vi "SLM.vi"() -> ()   [LabVIEW 2019]
uses:
  PCIe16LabVIEWSDK/Interface.dll
panel:
  out "Phase Image":u16[][](array[numeric])
  out "SLM":bool
  in  "Start SLM":bool
  out "Update SLM":bool
  out "PCIe16SDK Path":string
  out "Board ID":i32
  out "# of Boards":i32
  in  "SLM Image Path":path
  out "SLM Image":T1(plugin-control)
  out "Init.":bool
  in  "Stop":bool
types:
  T1 = typedef "IMAQ Image.ctl" = refnum<image>
  T2 = typedef "Image Type" = u32
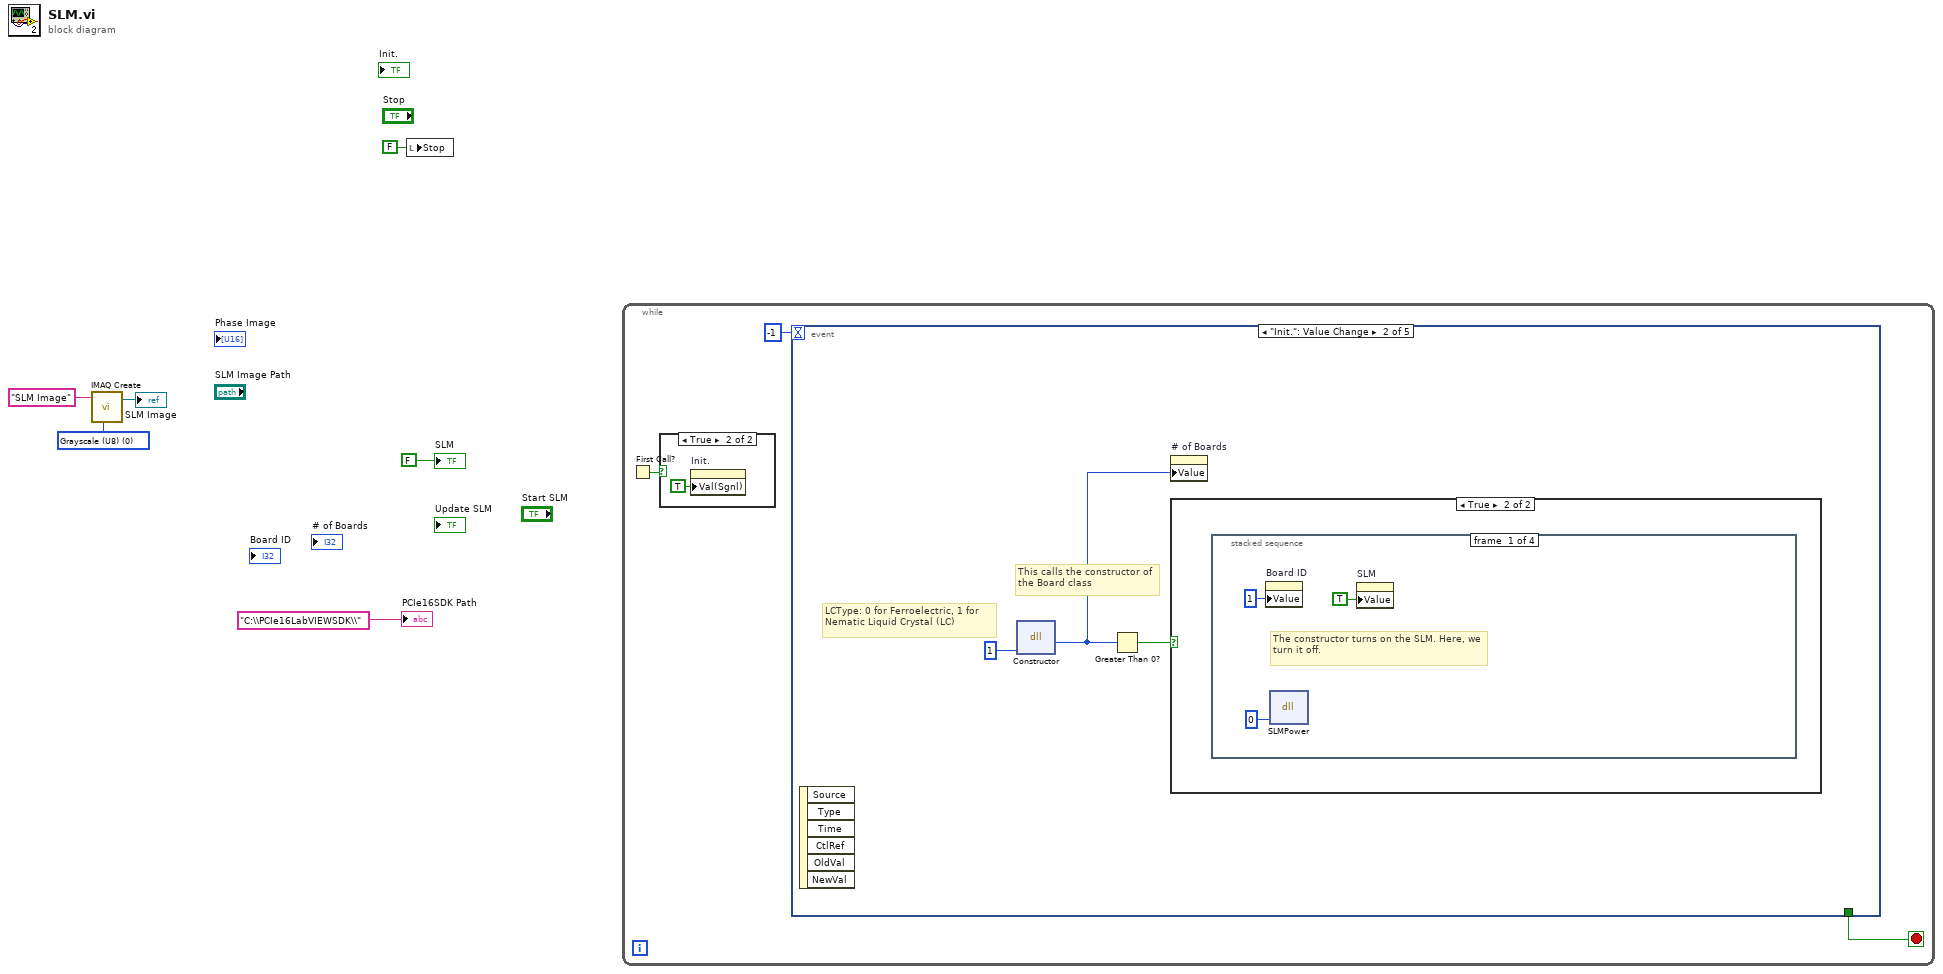
[diagram p0: block diagram]
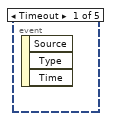
[diagram p3: hidden frame]
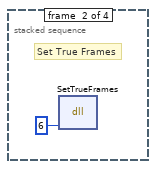
[diagram p5: hidden frame]
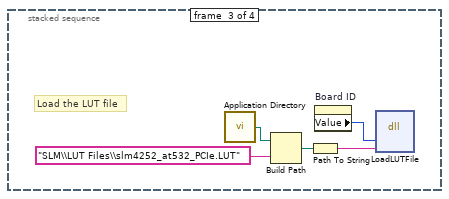
[diagram p6: hidden frame]
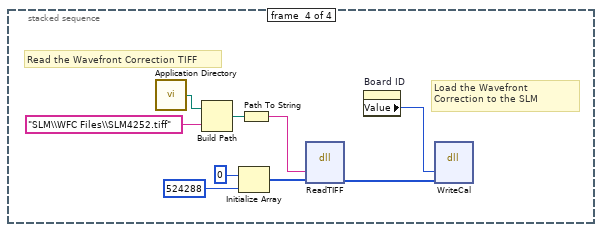
[diagram p7: hidden frame]
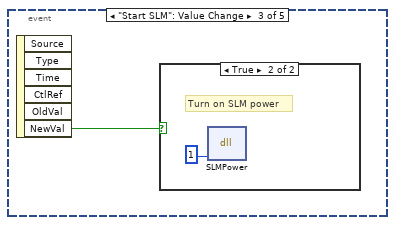
[diagram p8: hidden frame]
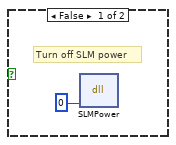
[diagram p9: hidden frame]
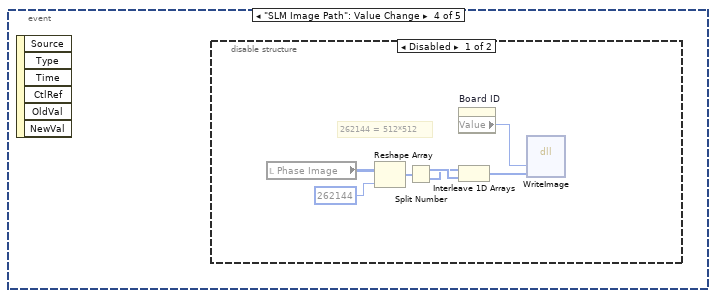
[diagram p10: hidden frame]
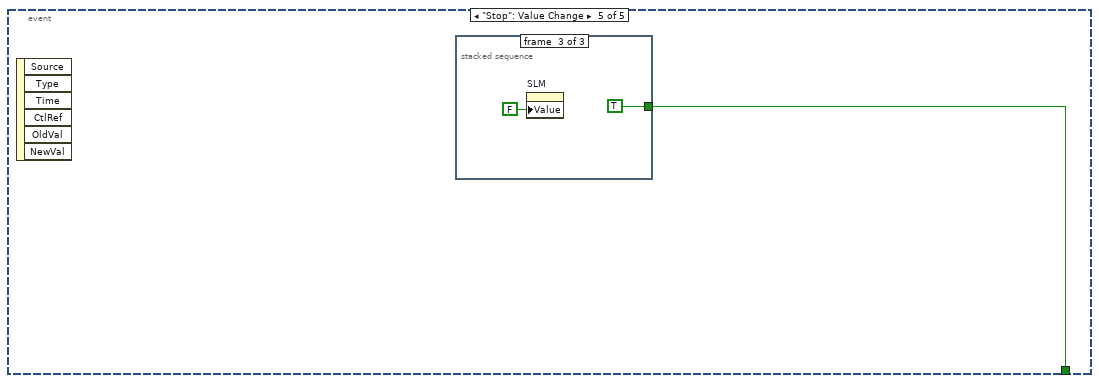
[diagram p12: hidden frame]
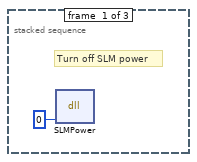
[diagram p13: hidden frame]
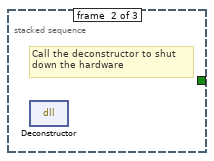
[diagram p14: hidden frame]
diagram:
  w3 = T2 0 items=["Grayscale (U8)", "Grayscale (I16)", "Grayscale (SGL)", "Complex (CSG)", "RGB (U32)", "HSL (U32)", "RGB (U64)", "Grayscale (U16)"] ("Image Type")
  n1 = call "IMAQ Create"("Image Name"="SLM Image", "Image Type"=w3) -> ("New Image"=→"SLM Image":T1)  [unwired: 3 in, 1 out]
  n2 = local write "Stop"(FALSE ("Stop")) -> ()
  n3 = while {
    stop <- w8 stop-if-true
    n4 = First Call?() -> (First Call?: T/F=w7:bool)
    n5 = case shown="True" w7 {
      frame False {
      }
      frame True {
        n6 = property on="Init." class="Bool (strict)"("Val(Sgnl)"=TRUE ("Value (Signaling)")) -> ()  [unwired: 2 in, 2 out]
      }
    }
    n7 = event shown="[1] \"Init.\": Value Change" {
      selector: _ -> [_ _ _ _ _]
      dyn-events: _ -> [_ _ _ _ _]
      timeout: -1 -> [_ _ _ _ _]
      tunnel: [_ _ _ _ w42] -> w8
      event Timeout {
        n8 = event-data() -> ()  [unwired: 1 in, 3 out]
      }
      event "Init.": Value Change {
        # "LCType: 0 for Ferroelectric, 1 for Nematic Liquid Crystal (LC)"
        # "This calls the constructor of the Board class"
        n9 = event-data() -> ()  [unwired: 1 in, 6 out]
        n10 = dll-call lib="C:/PCIe16LabVIEWSDK/Interface.dll" fn="Constructor"("LCType"=u8 1) -> ("return type"=w11:i32)  [unwired: 4 in, 2 out]
        n11 = Greater Than 0?(x=w11) -> (x > 0?=w13:bool)
        n12 = property on="# of Boards" class="DigNum (strict)"("Value"=w11) -> ()  [unwired: 2 in, 2 out]
        n13 = case shown="True" w13 {
          frame False {
          }
          frame True {
            n14 = stacked-sequence {
              frame #0 {
                # "The constructor turns on the SLM. Here, we turn it off."
                n15 = property on="Board ID" class="DigNum (strict)"("Value"=1 ("Board Number")) -> ()  [unwired: 2 in, 2 out]
                n16 = dll-call lib="C:/PCIe16LabVIEWSDK/Interface.dll" fn="SLMPower"("PowerState"=0) -> ()  [unwired: 5 in, 2 out]
                n17 = property on="SLM" class="Bool (strict)"("Value"=TRUE ("SLM")) -> ()  [unwired: 2 in, 2 out]
              }
              frame #1 {
                # "Set True Frames"
                n18 = dll-call lib="C:/PCIe16LabVIEWSDK/Interface.dll" fn="SetTrueFrames"("TrueFrames"=6) -> ()  [unwired: 5 in, 2 out]
              }
              frame #2 {
                # "Load the LUT file"
                n19 = call <vilib>:"Application Directory.vi"() -> ("Application Directory"=w20:path)
                n20 = Build Path(base path=w20, name or relative path="SLM\\LUT Files\\slm4252_at532_PCIe.LUT") -> (appended path=w21:path)
                n21 = Path To String(path=w21) -> (string=w18:string)
                n22 = property on="Board ID" class="DigNum (strict)"() -> ("Value"=w22:i32)  [unwired: 2 in, 2 out]
                n23 = dll-call lib="C:/PCIe16LabVIEWSDK/Interface.dll" fn="LoadLUTFile"("board"=w22, "LUTPath"=w18) -> ()  [unwired: 6 in, 2 out]
              }
              frame #3 {
                # "Read the Wavefront Correction TIFF"
                # "Load the Wavefront Correction to the SLM"
                n24 = call <vilib>:"Application Directory.vi"() -> ("Application Directory"=w28:path)
                n25 = Build Path(base path=w28, name or relative path="SLM\\WFC Files\\SLM4252.tiff") -> (appended path=w29:path)
                n26 = Initialize Array(u8 0, 524288) -> (w23:u8[])
                n27 = Path To String(path=w29) -> (string=w26:string)
                n28 = dll-call lib="C:/PCIe16LabVIEWSDK/Interface.dll" fn="ReadTIFF"("TiffPath"=w26, "Image"=w23) -> ("Image"=w31:u8[])  [unwired: 5 in, 2 out]
                n29 = property on="Board ID" class="DigNum (strict)"() -> ("Value"=w30:i32)  [unwired: 2 in, 2 out]
                n30 = dll-call lib="C:/PCIe16LabVIEWSDK/Interface.dll" fn="WriteCal"("board"=w30, "Image"=w31) -> ()  [unwired: 6 in, 2 out]
              }
            }
          }
        }
      }
      event "Start SLM": Value Change {
        n31 = event-data() -> ("NewVal"=w32:bool)  [unwired: 1 in, 5 out]
        n32 = case shown="True" w32 {
          frame False {
            # "Turn off SLM power"
            n33 = dll-call lib="C:/PCIe16LabVIEWSDK/Interface.dll" fn="SLMPower"("PowerState"=0) -> ()  [unwired: 5 in, 2 out]
          }
          frame True {
            # "Turn on SLM power"
            n34 = dll-call lib="C:/PCIe16LabVIEWSDK/Interface.dll" fn="SLMPower"("PowerState"=1) -> ()  [unwired: 5 in, 2 out]
          }
        }
      }
      event "SLM Image Path": Value Change {
        n35 = event-data() -> ()  [unwired: 1 in, 6 out]
        n36 = disable-structure shown="Disabled" {
          frame Disabled {
            # "262144 = 512*512"
            n37 = local read "Phase Image"() -> (w36:u16[][])
            n38 = Reshape Array(w36, 262144 ("dimension size")) -> (w38:u16[])
            n39 = Split Number(x=w38) -> (hi(x)=w41:u8[], lo(x)=w40:u8[])
            n40 = property on="Board ID" class="DigNum (strict)"() -> ("Value"=w37:i32)  [unwired: 2 in, 2 out]
            n41 = Interleave 1D Arrays(w40, w41) -> (w39:u8[])
            n42 = dll-call lib="C:/PCIe16LabVIEWSDK/Interface.dll" fn="WriteImage"("board"=w37, "Image"=w39) -> ()  [unwired: 6 in, 2 out]
          }
          frame Enabled {
          }
        }
      }
      event "Stop": Value Change {
        n43 = event-data() -> ()  [unwired: 1 in, 6 out]
        n44 = stacked-sequence {
          tunnel: [_ _ TRUE] -> w42
          frame #0 {
            # "Turn off SLM power"
            n45 = dll-call lib="C:/PCIe16LabVIEWSDK/Interface.dll" fn="SLMPower"("PowerState"=0) -> ()  [unwired: 5 in, 2 out]
          }
          frame #1 {
            # "Call the deconstructor to shut \ndown the hardware"
            n46 = dll-call lib="C:/PCIe16LabVIEWSDK/Interface.dll" fn="Deconstructor"() -> ()  [unwired: 4 in, 2 out]
          }
          frame #2 {
            n47 = property on="SLM" class="Bool (strict)"("Value"=FALSE ("SLM")) -> ()  [unwired: 2 in, 2 out]
          }
        }
      }
    }
  }
  "PCIe16SDK Path" <- "C:\\PCIe16LabVIEWSDK\\"
  "SLM" <- FALSE
